vi "计算方法调试工具.vi"() -> ()   [LabVIEW 2015, in "Logging.lvlib"]
uses:
  Logging.lvlib
  Measure/Measure Type.ctl
  <vilib>/Utility/file.llb/Read Delimited Spreadsheet (DBL).vi
panel:
  out "XY Graph 2":cluster{"Y":dbl[], "Y":dbl[]}[](graph) caption="XY图"
  out "波形图":dbl[](graph)
  out "XY Graph":cluster{"Y":dbl[], "Y":dbl[]}[](graph) caption="XY图"
  in  "计算":bool
  in  "测试类型":T1
  in  "文件路径":path
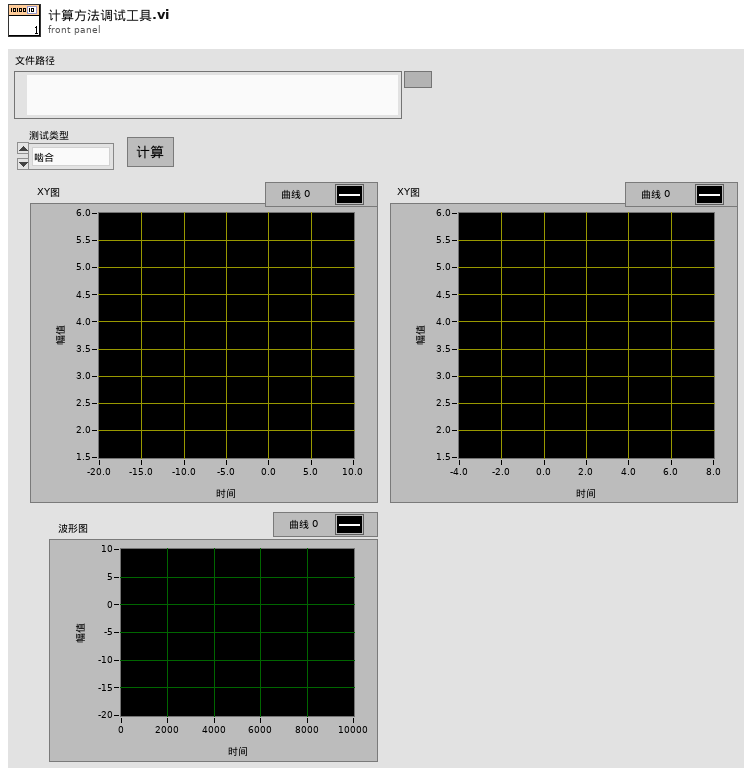
[diagram p1: front panel]
types:
  T1 = typedef "Measure Type.ctl" = enum16{"啮合", "退回", "功能", "力特性", "内泄漏", "分中", "对中"}
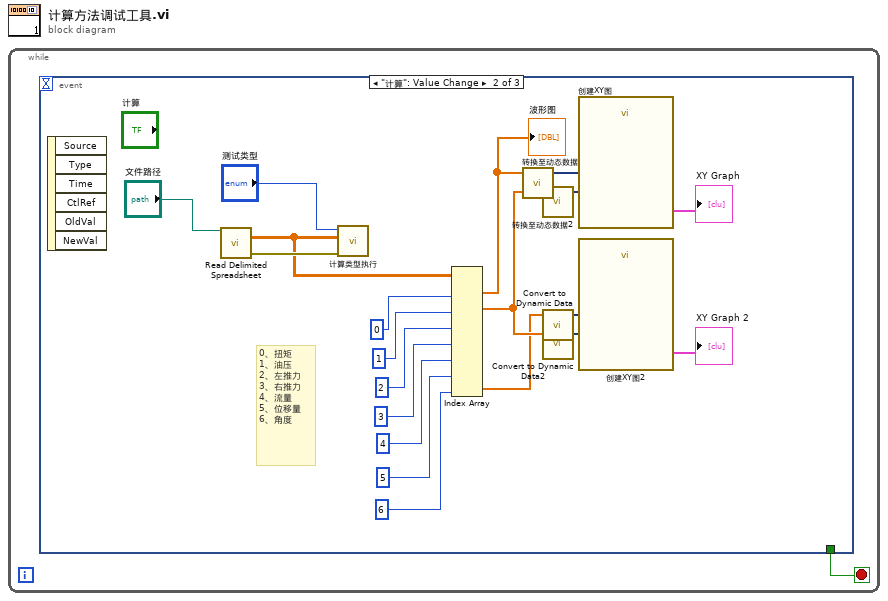
[diagram p0: block diagram]
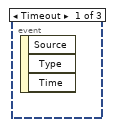
[diagram p2: hidden frame]
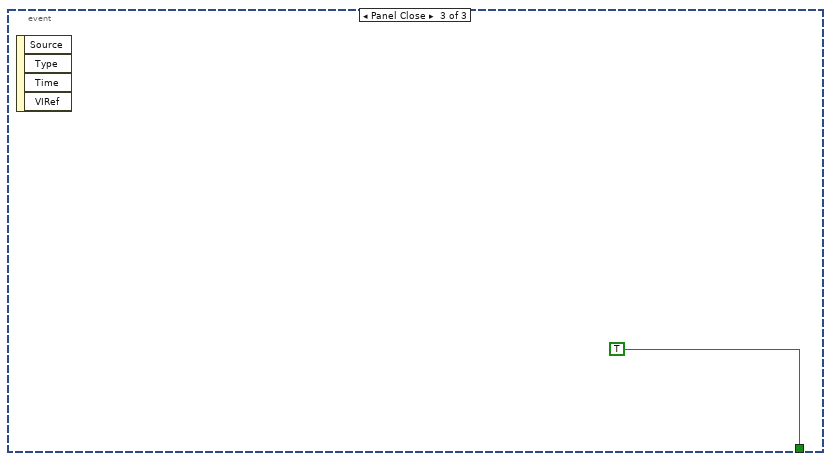
[diagram p3: hidden frame]
diagram:
  n1 = while {
    stop <- w1 stop-if-true
    n2 = event shown="[1] \"计算\": Value Change" {
      selector: _ -> [_ _ _]
      dyn-events: _ -> [_ _ _]
      timeout: _ -> [_ _ _]
      tunnel: [_ _ TRUE] -> w1
      event Timeout {
        n3 = event-data() -> ()  [unwired: 1 in, 3 out]
      }
      event "计算": Value Change {
        # "0、扭矩\n1、油压\n2、左推力\n3、右推力\n4、流量\n5、位移量\n6、角度"
        n4 = event-data() -> ()  [unwired: 1 in, 6 out]
        n5 = call-poly <vilib>:"Read Delimited Spreadsheet.vi"("file path (dialog if empty)"="文件路径") -> ("all rows"=w17:dbl[][], "error out"=w19:errorcluster)  [unwired: 9 in, 4 out]
        n6 = call "计算类型执行.vi"("error in (no error)"=w19, "信号数据"=w17, "计算类型"="测试类型") -> ()  [unwired: 8 in, 1 out]
        n7 = Index Array(array=w17, index (col) #1=0 ("禁用的索引 (列)"), index (col) #2=1 ("索引 (行)"), index (col) #3=2 ("索引 (行)"), index (col) #4=3 ("索引 (行)"), index (col) #5=4 ("索引 (行)"), index (col) #6=5 ("索引 (行)"), index (col) #7=6 ("index (col)")) -> (element #1=w14:dbl[], element #2=w5:dbl[], element #7=w2:dbl[])  [unwired: 7 in, 4 out]
        "波形图" <- w14
        n8 = call "转换至动态数据"("Array"=w14) -> ("Dynamic Data Type"=w16:dynamicdata)  [unwired: 3 in]
        n9 = call "转换至动态数据2"("Array"=w5) -> ("Dynamic Data Type"=w15:dynamicdata)  [unwired: 3 in]
        n10 = call "Convert to Dynamic Data"("Array"=w2) -> ("Dynamic Data Type"=w6:dynamicdata)  [unwired: 3 in]
        n11 = call "Convert to Dynamic Data2"("Array"=w5) -> ("Dynamic Data Type"=w4:dynamicdata)  [unwired: 3 in]
        n12 = call "创建XY图"("Y Input"=w15, "X Input"=w16) -> ("XY Graph"=→"XY Graph":cluster{"X":dbl[], "Y":dbl[]}[])  [unwired: 8 in, 1 out]
        n13 = call "创建XY图2"("Y Input"=w4, "X Input"=w6) -> ("XY Graph"=→"XY Graph 2":cluster{"X":dbl[], "Y":dbl[]}[])  [unwired: 8 in, 1 out]
      }
      event Panel Close {
        n14 = event-data() -> ()  [unwired: 1 in, 4 out]
      }
    }
  }
